vi "toml_api_file_read.vi"(8 "error in (no error)":errorcluster, 10 "operation (open or create)":T1(ring)=enum."open or create", 11 "resolved path":path) -> (0 "error out":errorcluster, 3 "text":string)   [LabVIEW 2017]
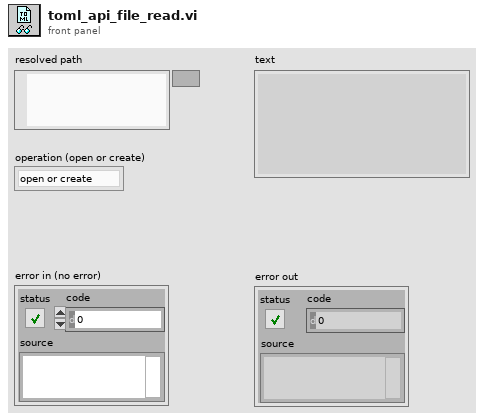
[diagram p1: front panel]
types:
  T1 = enum16{"open", "replace", "create", "open or create", "replace or create", "replace or create with confirmation"}
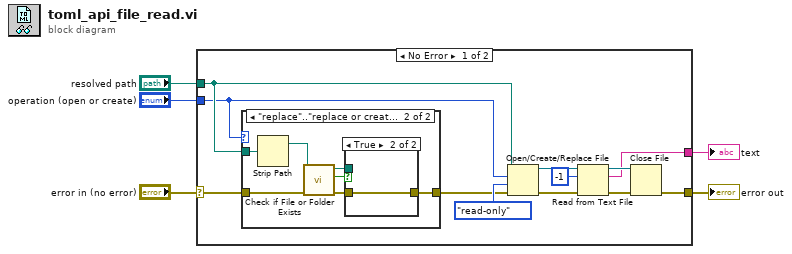
[diagram p0: block diagram]
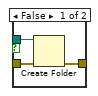
[diagram p3: hidden frame]
diagram:
  n1 = case shown="No Error" "error in (no error)" {
    selector: "error in (no error)" -> [w9 w30]
    tunnel: "resolved path" -> [w8 _]
    tunnel: [w13 _] -> w3
    tunnel: [w12 w30] -> w2
    tunnel: "operation (open or create)" -> [w6 _]
    frame No Error {
      n2 = case shown="\"replace\"..\"replace or create with confirmation\"" w6 {
        tunnel: w9 -> [w18 w25]
        tunnel: w8 -> [_ w23]
        tunnel: [w18 w21] -> w7
        frame "open" {
          # "don't create directory"
        }
        frame "replace".."replace or create with confirmation" {
          n3 = Strip Path(path=w23) -> (stripped path=w24:path)  [unwired: 1 out]
          n4 = call <vilib>:"Check if File or Folder Exists.vi"("error in (no error)"=w25, "path"=w24) -> ("error out"=w22:errorcluster, "file or folder exists?"=w19:bool, "dup path"=w20:path)  [unwired: 7 in]
          n5 = case shown="True" w19 {
            tunnel: w22 -> [w28 w29]
            tunnel: [w27 w29] -> w21
            tunnel: w20 -> [w26 _]
            frame False {
              n6 = Create Folder(path (use dialog)=w26, error in=w28) -> (error out=w27:errorcluster)  [unwired: 1 in, 2 out]
            }
            frame True {
            }
          }
        }
      }
      n7 = Open/Create/Replace File(file path (use dialog)=w8, error in=w7, operation (0:open)=w6, access (0:read/write)=enum16{"read/write", "read-only", "write-only"}."read-only") -> (refnum out=w16:refnum<file>, error out=w17:errorcluster)  [unwired: 2 in, 1 out]
      n8 = Read from Text File(file (use dialog)=w16, count=-1, error in=w17) -> (refnum out=w14:refnum<file>, text=w13:string, error out=w15:errorcluster)  [unwired: 1 in, 1 out]
      n9 = Close File(refnum=w14, error in=w15) -> (error out=w12:errorcluster)  [unwired: 1 out]
    }
    frame Error {
    }
  }
  "error out" <- w2
  "text" <- w3
